vi "Draw Wedge.vi"(4 "wheel frame angle (rad)":dbl, 6 "color":u32(colorbox)=12369084, 7 "picture info":T1={"picture size"={"Width"=500, "Height"=500}, "pixels per unit"=10.0}, 8 "steering angle range":T3={"min steering angle (rad)"=-3.14159, "max steering angle (rad)"=3.141592653589793}, 9 "radius":dbl, 10 "global wheel position":cluster{"x":dbl, "y":dbl}, 11 "picture in":picture) -> (3 "picture out":picture)   [LabVIEW 2017, in "NI_Robotics_Steering Picture.lvlib"]
uses:
  <vilib>/robotics/Utilities/Visualization/Steering Visualization/Steering Picture/NI_Robotics_Steering Picture.lvlib
  <vilib>/robotics/Steering/Steering Wheel/Steering Angle Range.ctl
  <vilib>/robotics/Utilities/Visualization/Steering Visualization/Steering Picture/Picture Info.ctl
  <vilib>/Utility/miscctls.llb/LVBoundsTypeDef.ctl
  <vilib>/Analysis/coordinate.llb/Angle Range (Degree).ctl
  <vilib>/Analysis/coordinate.llb/2D Cartesian Coordinate Rotation (Array).vi
  <vilib>/Analysis/coordinate.llb/Wrap Angle (scalar).vi
  <vilib>/Utility/AngleManip/Radians to Degrees (Scalar DBL).vi
  <vilib>/Utility/AngleManip/NI_AngleManipulation.lvlib
  <vilib>/Analysis/NI_AALPro.lvlib
  <vilib>/Analysis/NI_AAL_Angle.lvlib
  <vilib>/robotics/Steering/Steering Wheel/NI_Robotics_Steering Wheel.lvclass
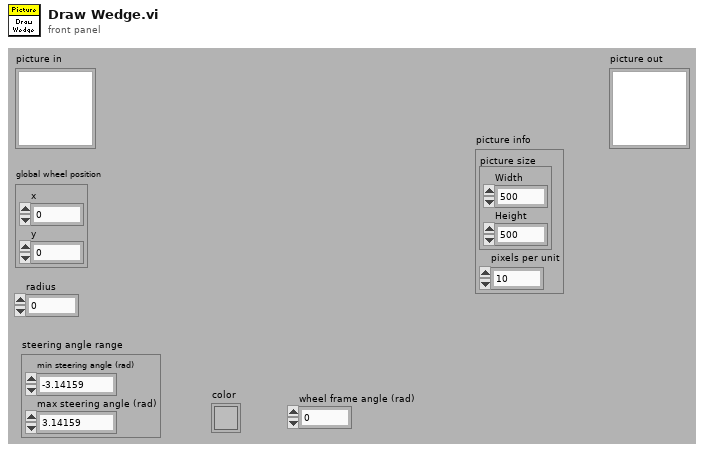
[diagram p1: front panel]
types:
  T1 = typedef "NI_Robotics_Steering Picture.lvlib/Picture Info.ctl" = cluster{"picture size":T2, "pixels per unit":dbl}
  T2 = typedef "LVBoundsTypeDef.ctl" = cluster{"Width":u32, "Height":u32}
  T3 = typedef "NI_Robotics_Steering Wheel.lvclass/Steering Angle Range.ctl" = cluster{"min steering angle (rad)":dbl, "max steering angle (rad)":dbl}
  T4 = typedef "NI_AAL_Angle.lvlib/Angle Range (Degree).ctl" = u16
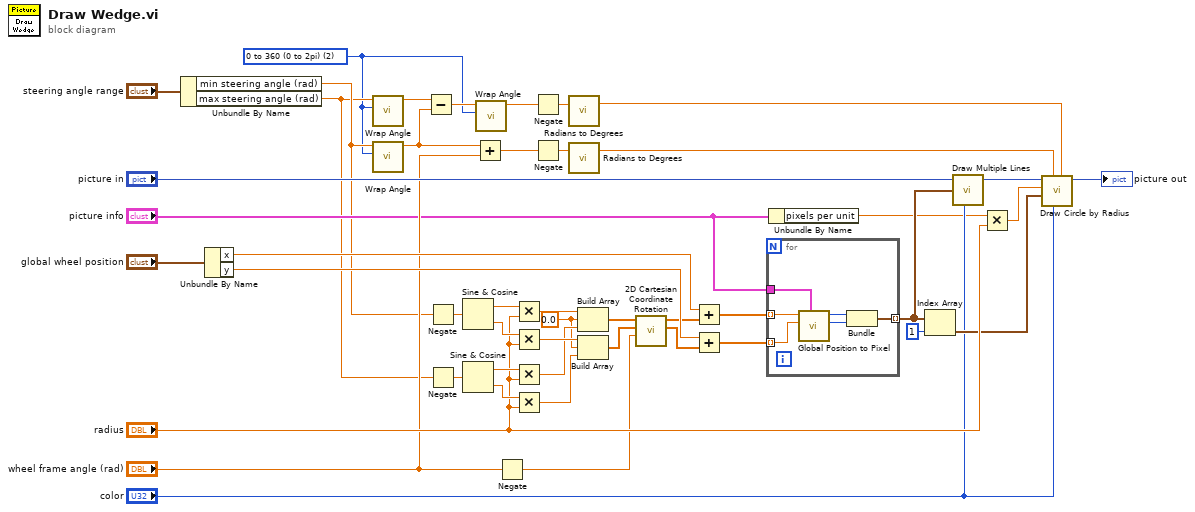
[diagram p0: block diagram]
diagram:
  w1 = T4 2 items=["none", "-180 to 180 (-pi to pi)", "0 to 360 (0 to 2pi)"] ("angle range")
  w32 = 0.0 ("element")
  n1 = Unbundle By Name("steering angle range") -> ("min steering angle (rad)"=w7:dbl, "max steering angle (rad)"=w5:dbl)
  n2 = Unbundle By Name("global wheel position") -> ("x"=w38:dbl, "y"=w37:dbl)
  n3 = call-poly <vilib>:"Wrap Angle.vi"("angle range"=w1, "angle in"=w5) -> ("angle out"=w4:dbl)  [unwired: 8 in, 1 out]
  n4 = call-poly <vilib>:"Wrap Angle.vi"("angle range"=w1, "angle in"=w7) -> ("angle out"=w6:dbl)  [unwired: 8 in, 1 out]
  n5 = Subtract(x=w4, y=w6) -> (x-y=w3:dbl)
  n6 = Negate(x=w7) -> (-x=w14:dbl)
  n7 = Negate(x=w5) -> (-x=w15:dbl)
  n8 = Sine & Cosine(0:w14) -> (1:w45:dbl, 2:w44:dbl)
  n9 = Sine & Cosine(0:w15) -> (1:w42:dbl, 2:w43:dbl)
  n10 = Add(x=w6, y="wheel frame angle (rad)") -> (x+y=w10:dbl)
  n11 = call-poly <vilib>:"Wrap Angle.vi"("angle range"=w1, "angle in"=w3) -> ("angle out"=w2:dbl)  [unwired: 8 in, 1 out]
  n12 = Negate(x="wheel frame angle (rad)") -> (-x=w18:dbl)
  n13 = Multiply(x=w45, y="radius") -> (x*y=w41:dbl)
  n14 = Multiply(x=w44, y="radius") -> (x*y=w40:dbl)
  n15 = Multiply(x=w42, y="radius") -> (x*y=w33:dbl)
  n16 = Multiply(x=w43, y="radius") -> (x*y=w34:dbl)
  n17 = Negate(x=w2) -> (-x=w12:dbl)
  n18 = Negate(x=w10) -> (-x=w13:dbl)
  n19 = call-poly <vilib>:"Radians to Degrees.vi"("angle (rad)"=w12) -> ("angle (deg)"=w16:dbl)  [unwired: 2 in]
  n20 = call-poly <vilib>:"Radians to Degrees.vi"("angle (rad)"=w13) -> ("angle (deg)"=w17:dbl)  [unwired: 2 in]
  n21 = Build Array(w41, w32, w33) -> (w22:dbl[])
  n22 = Build Array(w40, w32, w34) -> (w20:dbl[])
  n23 = call-poly <vilib>:"2D Cartesian Coordinate Rotation.vi"("theta"=w18, "Y"=w20, "X"=w22) -> ("Y Out"=w19:dbl[], "X Out"=w21:dbl[])  [unwired: 6 in, 1 out]
  n24 = Add(x=w38, y=w21) -> (x+y=w36:dbl[])
  n25 = Add(x=w37, y=w19) -> (x+y=w35:dbl[])
  n26 = for {
    tunnel: w36 -> [w52] mode=indexing
    tunnel: w35 -> [w51] mode=indexing
    tunnel: [w48] -> w27 mode=indexing
    tunnel: "picture info" -> [w47]
    n27 = call <vilib>:"Global Position to Pixel.vi"("picture info"=w47, "global y"=w51, "global x"=w52) -> ("pixel y"=w49:i16, "pixel x"=w50:i16)  [unwired: 7 in]
    n28 = Bundle("pixel x"=w50, "pixel y"=w49) -> (w48:cluster{"pixel x":i16, "pixel y":i16})  [unwired: 1 in]
  }
  n29 = Unbundle By Name("picture info") -> ("pixels per unit"=w8:dbl)
  n30 = Index Array(array=w27, index=1) -> (element=w25:cluster{"pixel x":i16, "pixel y":i16})
  n31 = call <vilib>:"Draw Multiple Lines.vi"("picture"="picture in", "line endpoints"=w27, "color(black)"="color") -> ("new picture"=w29:picture)  [unwired: 6 in]
  n32 = Multiply(x=w8, y="radius") -> (x*y=w28:dbl)
  n33 = call <vilib>:"Draw Circle by Radius.vi"("arc size(360)"=w16, "color(black)"="color", "start angle(0)"=w17, "pixel center"=w25, "radius"=w28, "picture"=w29) -> ("new picture"=→"picture out":picture)  [unwired: 5 in]
